vi "Stepper Mover Text In.vi"(1 "command text in":string[](array[string])=["N/A", "Magent PS", "N/A", "Set Field", "Set Field to 2.0000E+0 @ 0.0000T /min, no wait , extra 0 sec wait", "N/A", "N/A", "", "1", "0", "N/A", "2.000000", "0.000000", "N/A", "N/A", "N/A", "N/A", "N/A", "N/A", "N/A", "N/A", "N/A", "N/A", "N/A", "N/A", "N/A", "N/A", "N/A", "N/A", "N/A", "N/A", "N/A", "N/A", "N/A"]) -> (0 "Stepper Mover":T1={"extra wait"=0, "Stepper Value"=1e-09, "Top or Bottom"=enum."Move to Top Position (deg)"} {"extra wait" min=0; "Stepper Value" format="%#.7e"})   [LabVIEW 2020]
uses:
  Stepper Mover.ctl
panel:
  out "Numeric":i32
  # "Stepper Mover"
  # "(Stepper Mover.vi needs to be open before using this program)"
  # "Value"
  # "seconds"
  # "AND wait extra"
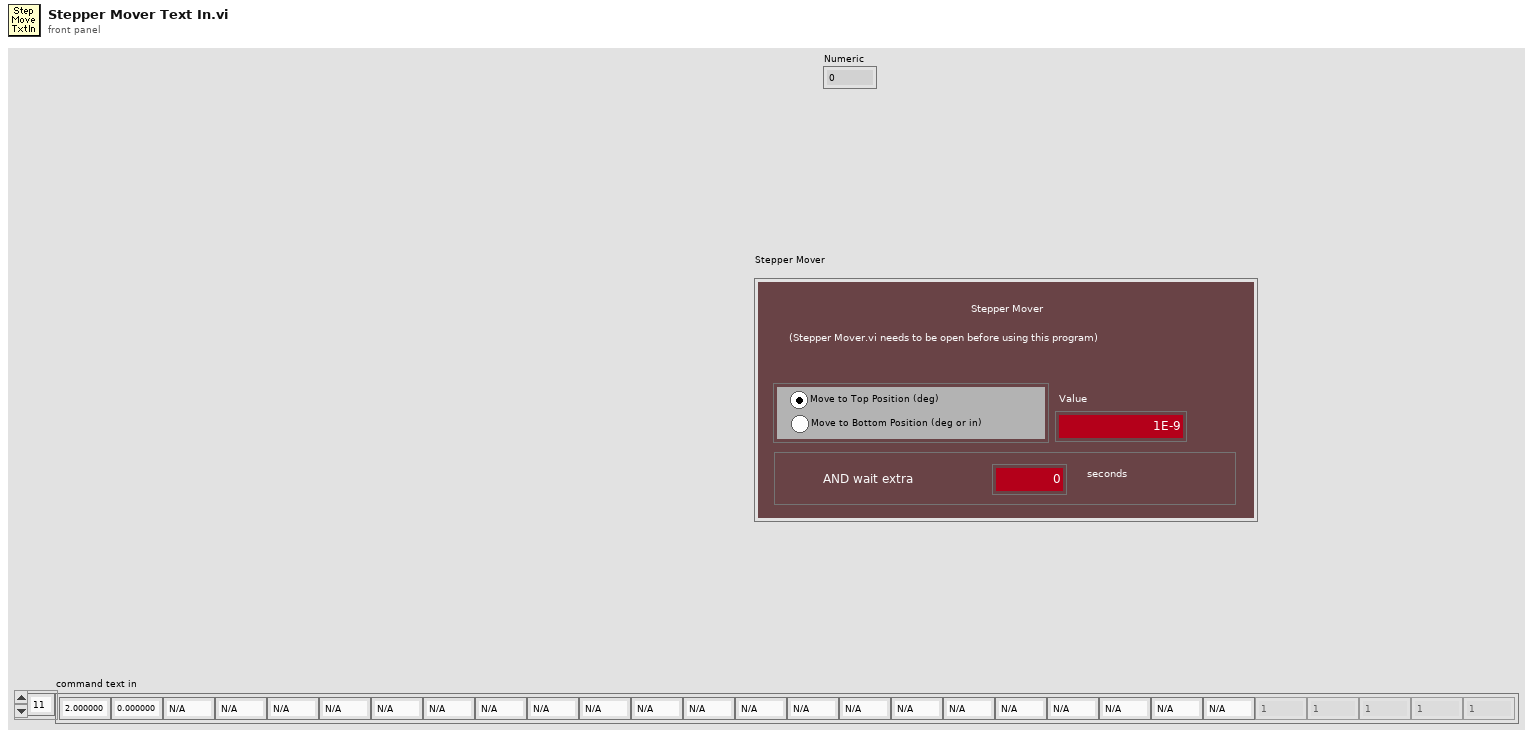
[diagram p1: front panel]
types:
  T1 = typedef "Stepper Mover.ctl" = cluster{"extra wait":i32, "Stepper Value":dbl, "Top or Bottom":enum32{"Move to Top Position (deg)", "Move to Bottom Position (deg or in)"}}
  T2 = cluster{"command text in[0]":string, "command text in[1]":string, "command text in[2]":string, "command text in[3]":string, "command text in[4]":string, "command text in[5]":string, "command text in[6]":string, "command text in[7]":string, "command text in[8]":string, "command text in[9]":string, "command text in[10]":string, "command text in[11]":string, "command text in[12]":string, "command text in[13]":string, "command text in[14]":string, "command text in[15]":string, "command text in[16]":string, "command text in[17]":string, "command text in[18]":string, "command text in[19]":string, "command text in[20]":string, "command text in[21]":string, "command text in[22]":string, "command text in[23]":string, "command text in[24]":string, "command text in[25]":string}
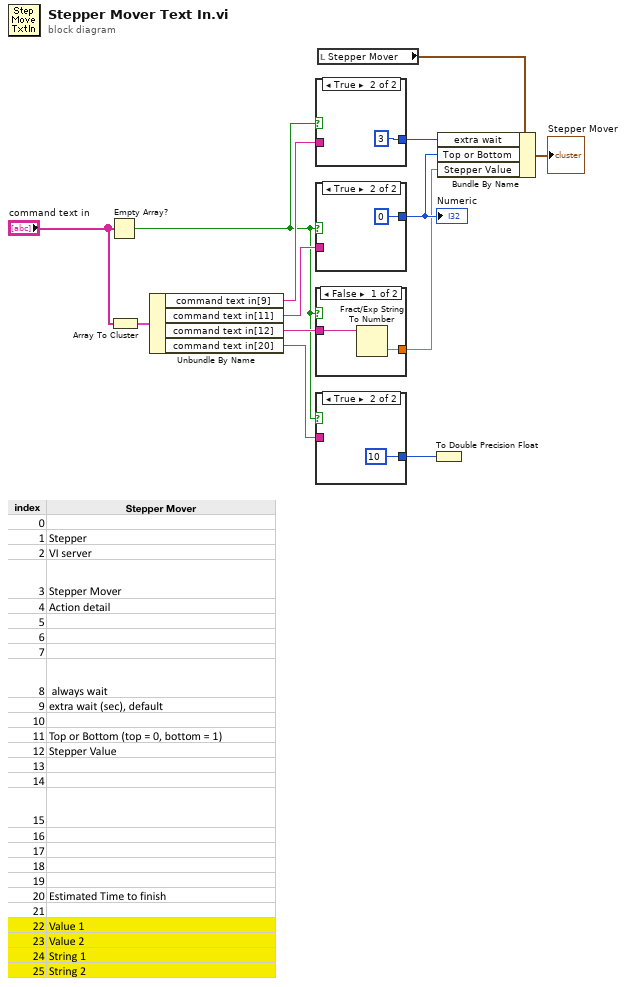
[diagram p0: block diagram]
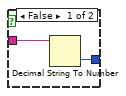
[diagram p2: hidden frame]
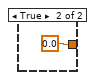
[diagram p3: hidden frame]
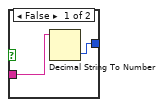
[diagram p4: hidden frame]
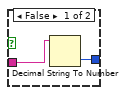
[diagram p5: hidden frame]
diagram:
  n1 = Empty Array?(array="command text in") -> (empty?=w1:bool)
  n2 = Array To Cluster(array="command text in") -> (cluster=w13:T2)
  n3 = Unbundle By Name(w13) -> ("command text in[9]"=w11:string, "command text in[11]"=w10:string, "command text in[12]"=w9:string, "command text in[20]"=w2:string)
  n4 = case shown="True" w1 {
    tunnel: w11 -> [w15 _]
    tunnel: [w14 u16 3 ("Value (Signaling)")] -> w6
    frame False {
      n5 = Decimal String To Number(string=w15) -> (number=w14:i32)  [unwired: 2 in, 1 out]
    }
    frame True {
    }
  }
  n6 = case shown="True" w1 {
    tunnel: w10 -> [w18 _]
    tunnel: [w17 0] -> w5
    frame False {
      n7 = Decimal String To Number(string=w18) -> (number=w17:i32)  [unwired: 2 in, 1 out]
    }
    frame True {
    }
  }
  "Numeric" <- w5
  n8 = case shown="False" w1 {
    tunnel: w9 -> [w20 _]
    tunnel: [w21 0.0] -> w4
    frame False {
      n9 = Fract/Exp String To Number(string=w20) -> (number=w21:dbl)  [unwired: 3 in, 1 out]
    }
    frame True {
    }
  }
  n10 = case shown="True" w1 {
    tunnel: w2 -> [w24 _]
    tunnel: [w23 10] -> w3
    frame False {
      n11 = Decimal String To Number(string=w24) -> (number=w23:i32)  [unwired: 2 in, 1 out]
    }
    frame True {
    }
  }
  n12 = local read "Stepper Mover"() -> (w8:T1)
  n13 = To Double Precision Float(number=w3) -> ()  [unwired: 1 out]
  n14 = Bundle By Name(cluster=w8, "extra wait"=w6, "Top or Bottom"=w5, "Stepper Value"=w4) -> (→"Stepper Mover":T1)
